vi "assign.vi"(8 "error in (no error)":errorcluster, 9 "value":variant, 10 "key chain":string[](array[string]), 11 "Map in":refnum<class "Map.lvclass">) -> (0 "error out":errorcluster, 3 "Map out":refnum<class "Map.lvclass">)   [LabVIEW 2010, in "Map.lvclass"]
doc: "This method sets the value for a given position in a map. The position is specified by the key array. \nFor a nested map, the key array contains all keys from root down to the desired position. If the key array refers to non-existing intermediary nodes, these are created on the fly. \nFor a non-nested map, simply provide an array with a single key value."
uses:
  Map.lvclass
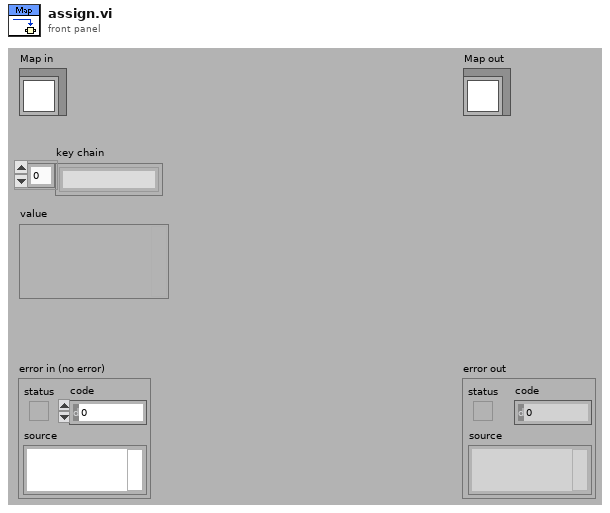
[diagram p1: front panel]
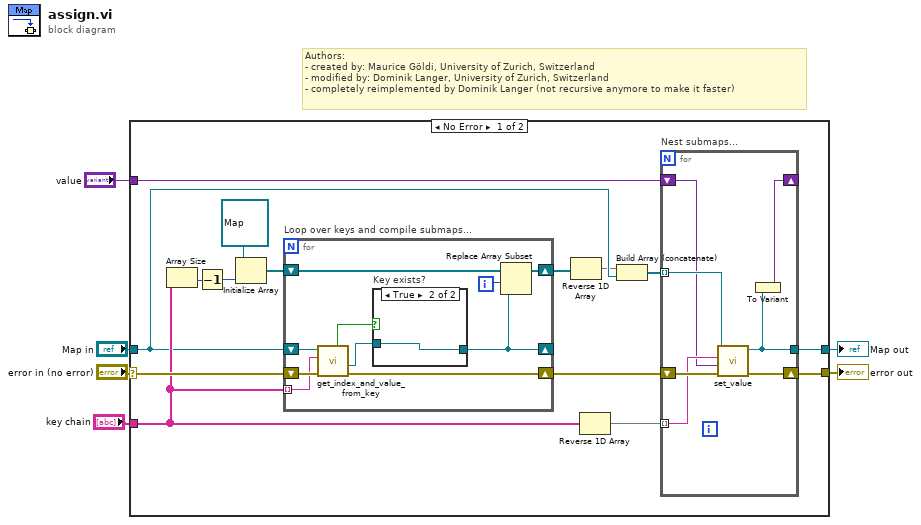
[diagram p0: block diagram]
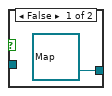
[diagram p2: hidden frame]
diagram:
  # "Authors: \n- created by: Maurice Göldi, University of Zurich, Switzerland\n- modified by: Dominik Langer, University of Zurich, Switzerland\n- completely reimplemented by Dominik Langer (not recursive anymore to make it faster)"
  n1 = case shown="No Error" "error in (no error)" {
    selector: "error in (no error)" -> [w21 w42]
    tunnel: [w14 w42] -> w5
    tunnel: [w10 w41] -> w3
    tunnel: "Map in" -> [w9 w41]
    tunnel: "key chain" -> [w12 _]
    tunnel: "value" -> [w13 _]
    frame No Error {
      n2 = Array Size(array=w12) -> (size(s)=w18:i32)
      n3 = Decrement(x=w18) -> (x-1=w16:i32)
      n4 = Initialize Array(refnum<class "Map.lvclass"> refnum ("Map.lvclass"), w16) -> (w19:refnum<class "Map.lvclass">[])
      n5 = for "Loop over keys and compile submaps..." {
        tunnel: w12 -> [w30] mode=indexing
        shift-right: [w33] -> w17
        shift-left: w21 -> [w38]
        shift-right: [w31] -> _
        shift-left: w9 -> [w32]
        shift-right: [w36] -> w15
        shift-left: w19 -> [w37]
        i -> [w29]
        n6 = call "get_index_and_value_from_key.vi"("error in (no error)"=w38, "key"=w30, "Map.lvclass in"=w32) -> ("error out"=w33:errorcluster, "submap"=w34:refnum<class "Map.lvclass">, "key exists?"=w35:bool)  [unwired: 6 out]
        n7 = case "Key exists?" shown="True" w35 {
          tunnel: w34 -> [_ w40]
          tunnel: [refnum<class "Map.lvclass"> refnum ("Map.lvclass") w40] -> w31
          frame False {
          }
          frame True {
          }
        }
        n8 = Replace Array Subset(array=w37, new element=w31, index=w29) -> (w36:refnum<class "Map.lvclass">[])
      }
      n9 = Reverse 1D Array(array=w15) -> (reversed array=w8:refnum<class "Map.lvclass">[])
      n10 = Reverse 1D Array(array=w12) -> (reversed array=w11:string[])
      n11 = Build Array (concatenate)(w8, w9) -> (w7:refnum<class "Map.lvclass">[])
      n12 = for "Nest submaps..." {
        shift-right: [w26] -> w14
        shift-left: w17 -> [w28]
        tunnel: w11 -> [w27] mode=indexing
        shift-right: [w24] -> _
        shift-left: w13 -> [w23]
        tunnel: w7 -> [w25] mode=indexing
        tunnel: [w22] -> w10
        n13 = call "set_value.vi"("error in (no error)"=w28, "value"=w23, "key"=w27, "Map.lvclass in"=w25) -> ("error out"=w26:errorcluster, "Map.lvclass out"=w22:refnum<class "Map.lvclass">)  [unwired: 6 out]
        n14 = To Variant(anything=w22) -> (Variant=w24:variant)
      }
    }
    frame Error {
    }
  }
  "error out" <- w5
  "Map out" <- w3
